vi "SoftSerial ESP8266 Tartget.vi"   [LabVIEW 2014]
doc: "The Serial - Monitoring GUI example shows best practices for a remote monitoring system with two VIs, one running on a host PC and the other running embedded in the Arduino compatible target. The example includes two-way serial communication between the host PC VI and the Arduino compatible target VI. This is the target VI taht generates a point by point sine wave that is charted by the host PC VI, writes the sine wave data points to the serial port and monitors the serial port for a potential pause/resume command to be sent by the host PC VI."
uses:
  <vilib>/Aledyne-TSXperts/Arduino Compatible Compiler for LabVIEW/Code Generator/Arduino APIs/Digital/PinDirection.ctl
  <vilib>/Aledyne-TSXperts/Arduino Compatible Compiler for LabVIEW/Arduino Compatible Compiler for LabVIEW.lvlib
  QwaveSys_ESP8266/QwaveSys_ESP8266.lvlib
types:
  T1 = typedef "Arduino Compatible Compiler for LabVIEW.lvlib/PinDirection.ctl" = enum16{" INPUT", "OUTPUT", " INPUT_PULLUP"}
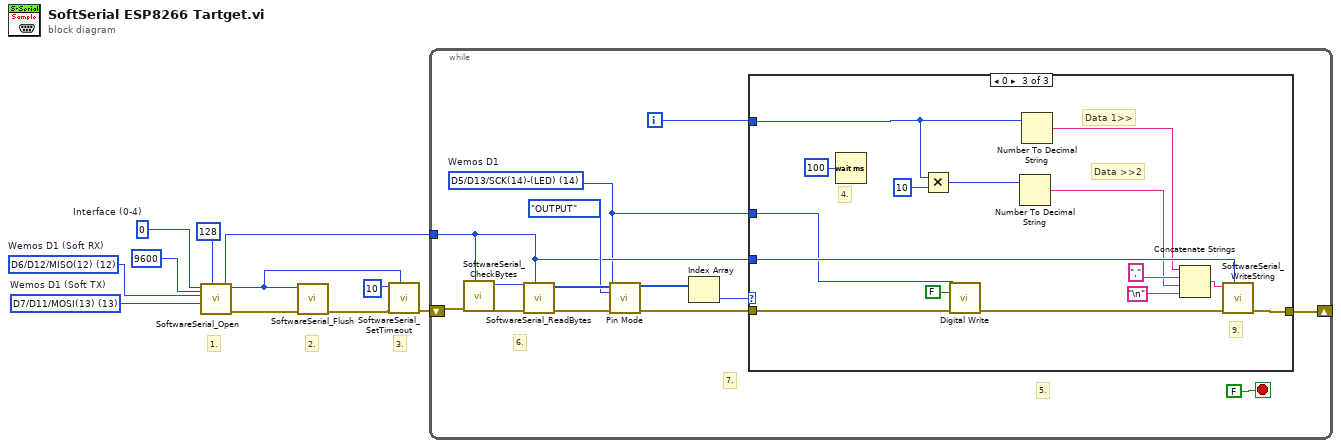
[diagram p0: block diagram]
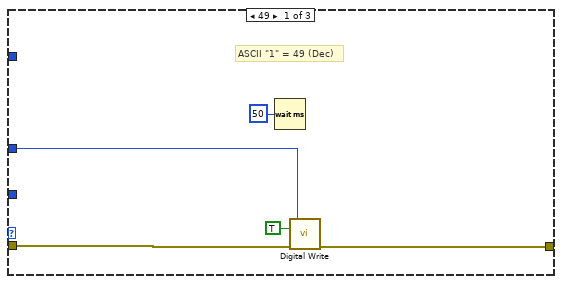
[diagram p2: hidden frame]
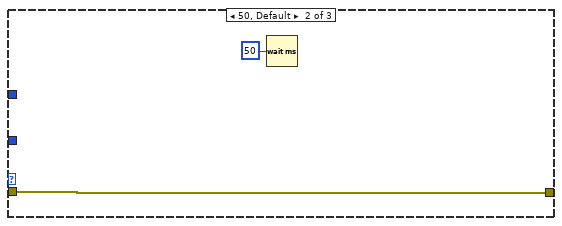
[diagram p3: hidden frame]
diagram:
  w1 = u8 13 items=["D0-RX(3)"=3, "D1-TX(1)"=1, "D2(16)"=16, "D3/D15/SCL(5)"=5, "D4/D14/SDA(4)"=4, "D5/D13/SCK(14)-(LED)"=14, "D6/D12/MISO(12)"=12, "D7/D11/MOSI(13)"=13, "D8(0)"=0, "D9/TX1(2)"=2, "D10/SS (15)"=15, "ADC0,(17)"=17]  # Wemos D1 (Soft TX)
  w2 = u8 12 items=["D0-RX(3)"=3, "D1-TX(1)"=1, "D2(16)"=16, "D3/D15/SCL(5)"=5, "D4/D14/SDA(4)"=4, "D5/D13/SCK(14)-(LED)"=14, "D6/D12/MISO(12)"=12, "D7/D11/MOSI(13)"=13, "D8(0)"=0, "D9/TX1(2)"=2, "D10/SS (15)"=15, "ADC0,(17)"=17]  # Wemos D1 (Soft RX)
  w3 = u8 0  # Interface (0-4)
  # "3."
  # "2."
  # "1."
  n1 = call "SoftwareSerial_Open.vi"("Speed"=u32 9600, "Buffer"=u8 128, "Tx"=w1, "Rx"=w2, "Interface (0-4)"=w3) -> ("error out"=w9:errorcluster, "Instance"=w7:u8)  [unwired: 5 in]
  n2 = call "SoftwareSerial_Flush.vi"("Instance"=w7, "error in (no error)"=w9) -> ("error out"=w8:errorcluster)  [unwired: 9 in]
  n3 = call "SoftwareSerial_SetTimeout.vi"("Instance"=w7, "error in (no error)"=w8, "Timeout (ms)"=10) -> ("error out"=w5:errorcluster)  [unwired: 8 in]
  n4 = while {
    tunnel: w7 -> [w12]
    shift-right: [w19] -> _
    shift-left: w5 -> [w15]
    i -> [w20]
    stop <- FALSE stop-if-true
    w11 = u8 14 items=["D0-RX(3)"=3, "D1-TX(1)"=1, "D2(16)"=16, "D3/D15/SCL(5)"=5, "D4/D14/SDA(4)"=4, "D5/D13/SCK(14)-(LED)"=14, "D6/D12/MISO(12)"=12, "D7/D11/MOSI(13)"=13, "D8(0)"=0, "D9/TX1(2)"=2, "D10/SS (15)"=15, "ADC0,(17)"=17]  # Wemos D1
    # "7."
    # "6."
    # "5."
    n5 = call "SoftwareSerial_CheckBytes.vi"("Instance"=w12, "error in (no error)"=w15) -> ("error out"=w14:errorcluster, "Bytes"=w13:i32)  [unwired: 8 in]
    n6 = call "SoftwareSerial_ReadBytes.vi"("Instance"=w12, "error in (no error)"=w14, "Length"=w13) -> ("error out"=w17:errorcluster, "Data"=w22:u8[])  [unwired: 6 in, 1 out]
    n7 = call <vilib>:"Pin Mode.vi"("pin"=w11, "direction"=PinDirection."OUTPUT", "error in (no error)"=w17) -> ("error out"=w16:errorcluster)  [unwired: 12 in]
    n8 = Index Array(array=w22) -> (element=w21:u8)  [unwired: 1 in]
    n9 = case shown="0" w21 {
      tunnel: [w26 w29 w45] -> w19
      tunnel: w16 -> [w27 w29 w34]
      tunnel: w12 -> [_ _ w44]
      tunnel: w20 -> [_ _ w38]
      tunnel: w11 -> [w25 _ w33]
      frame 49 {
        # "ASCII \"1\" = 49 (Dec)"
        n10 = Wait (ms)(milliseconds to wait=u32 50) -> ()  [unwired: 1 out]
        n11 = call <vilib>:"Digital Write.vi"("pin"=w25, "state"=TRUE, "error in (no error)"=w27) -> ("error out"=w26:errorcluster)  [unwired: 12 in]
      }
      frame 50, Default {
        n12 = Wait (ms)(milliseconds to wait=u32 50) -> ()  [unwired: 1 out]
      }
      frame 0 {
        # "Data >>2"
        # "Data 1>>"
        # "4."
        # "9."
        n13 = Wait (ms)(milliseconds to wait=u32 100) -> ()  [unwired: 1 out]
        n14 = Multiply(x=w38, y=10) -> (x*y=w32:i32)
        n15 = call <vilib>:"Digital Write.vi"("pin"=w33, "state"=FALSE, "error in (no error)"=w34) -> ("error out"=w36:errorcluster)  [unwired: 12 in]
        n16 = Number To Decimal String(number=w32) -> (decimal integer string=w31:string)  [unwired: 1 in]
        n17 = Number To Decimal String(number=w38) -> (decimal integer string=w39:string)  [unwired: 1 in]
        n18 = Concatenate Strings(w39, ",", w31, "\n" ("Line Feed Constant")) -> (w42:string)
        n19 = call "SoftwareSerial_WriteString.vi"("Instance"=w44, "error in (no error)"=w36, "String"=w42) -> ("error out"=w45:errorcluster)  [unwired: 8 in]
      }
    }
  }
